vi "TCP-unpack.vi"(11 "TCP RX in":string) -> (0 "Success":bool, 1 "TCP data":string, 2 "bytecount":i32, 3 "TCP RX out (rest)":string, 5 "CountOK":bool)   [LabVIEW 2020, in "Sgraph_lib_V1.lvlib"]
uses:
  Builds/Sgraph_lib_V1.lvlib
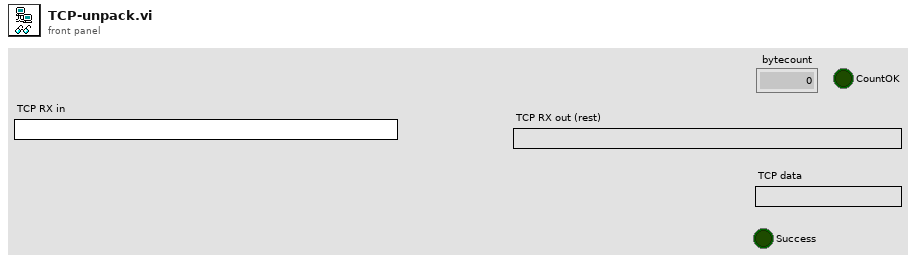
[diagram p1: front panel]
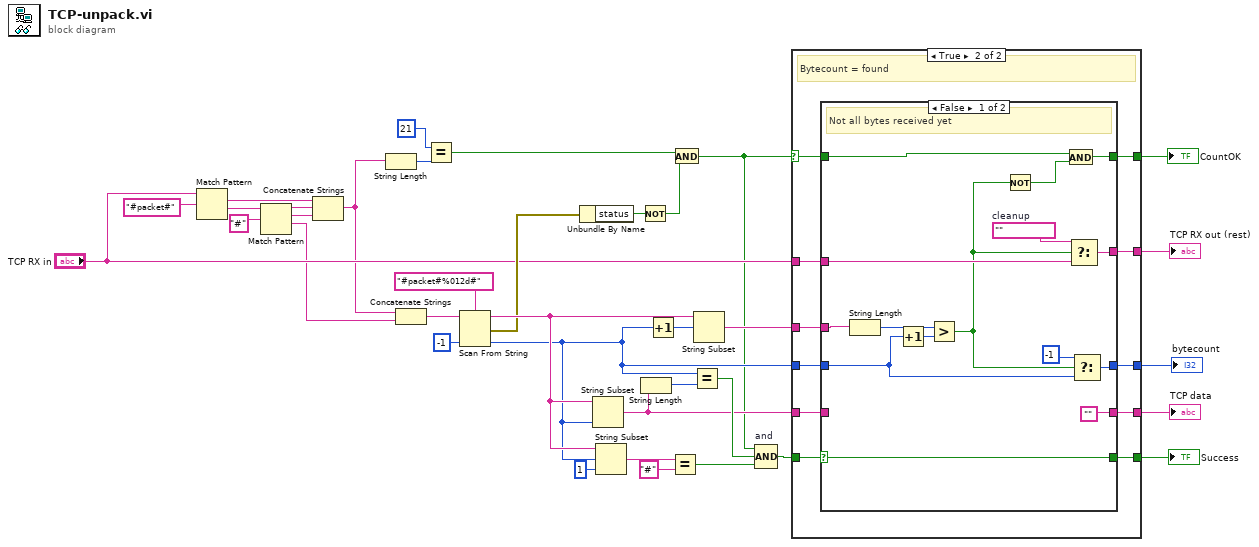
[diagram p0: block diagram]
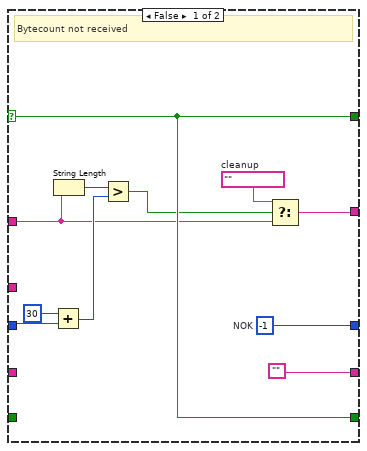
[diagram p2: hidden frame]
diagram:
  n1 = Match Pattern(string="TCP RX in", regular expression="#packet#" ("format string")) -> (match substring=w21:string, after substring=w23:string)  [unwired: 1 in, 2 out]
  n2 = Match Pattern(string=w23, regular expression="#" ("format string")) -> (before substring=w20:string, match substring=w19:string, after substring=w2:string)  [unwired: 1 in, 1 out]
  n3 = Concatenate Strings(w21, w20, w19) -> (w3:string)
  n4 = String Length(string=w3) -> (length=w18:i32)
  n5 = Concatenate Strings(w3, w2) -> (w1:string)
  n6 = Equal?(x=21, y=w18) -> (x = y?=w15:bool)
  n7 = Scan From String(format string="#packet#%012d#", input string=w1, default 1=-1 ("default value 1")) -> (remaining string=w31:string, error out=w27:errorcluster, output 1=w7:i32)  [unwired: 2 in, 1 out]
  n8 = Unbundle By Name(w27) -> ("status"=w26:bool)
  n9 = String Subset(string=w31, length (rest)=w7) -> (substring=w5:string)  [unwired: 1 in]
  n10 = String Subset(string=w31, offset (0)=w7, length (rest)=1 ("length (rest)")) -> (substring=w33:string)
  n11 = Not(x=w26) -> (.not. x?=w16:bool)
  n12 = String Length(string=w5) -> (length=w34:i32)
  n13 = Increment(x=w7) -> (x+1=w30:i32)
  n14 = Equal?(x=w33, y="#") -> (x = y?=w28:bool)
  n15 = And(x=w15, y=w16) -> (x .and. y?=w4:bool)
  n16 = Equal?(x=w7, y=w34) -> (x = y?=w29:bool)
  n17 = String Subset(string=w31, offset (0)=w30) -> (substring=w6:string)  [unwired: 1 in]
  n18 = Compound Arithmetic op=AND "and"(w4, w29, w28) -> (w8:bool)
  n19 = case shown="True" w4 {
    selector: w4 -> [w45 w49]
    tunnel: [w45 w48] -> w14
    tunnel: [w47 w52] -> w13
    tunnel: "TCP RX in" -> [w39 w56]
    tunnel: [w40 w55] -> w11
    tunnel: ["" w54] -> w10
    tunnel: [w45 w57] -> w9
    tunnel: w8 -> [_ w58]
    tunnel: w7 -> [w43 w53]
    tunnel: w6 -> [_ w51]
    tunnel: w5 -> [_ w50]
    frame False {
      w38 = ""  # cleanup
      w47 = -1  # NOK
      # "Bytecount not received"
      n20 = Add(x=30, y=w43) -> (x+y=w41:i32)
      n21 = String Length(string=w39) -> (length=w44:i32)
      n22 = Greater?(x=w44, y=w41) -> (0:w37:bool)
      n23 = Select(t=w38, s=w37, f=w39) -> (s? t:f=w40:string)
    }
    frame True {
      # "Bytecount = found"
      n24 = case shown="False" w58 {
        selector: w58 -> [w73 w78]
        tunnel: [w73 w78] -> w57
        tunnel: w56 -> [w68 _]
        tunnel: [w67 w77] -> w55
        tunnel: ["" w75] -> w54
        tunnel: w53 -> [w61 w76]
        tunnel: [w60 w76] -> w52
        tunnel: w51 -> [w71 w77]
        tunnel: w50 -> [_ w75]
        tunnel: w49 -> [w65 w74]
        tunnel: [w64 w74] -> w48
        frame False {
          w66 = ""  # cleanup
          # "Not all bytes received yet"
          n25 = String Length(string=w71) -> (length=w70:i32)
          n26 = Increment(x=w61) -> (x+1=w69:i32)
          n27 = Greater?(x=w70, y=w69) -> (0:w62:bool)
          n28 = Not(x=w62) -> (.not. x?=w63:bool)
          n29 = And(x=w65, y=w63) -> (x .and. y?=w64:bool)
          n30 = Select(t=w66, s=w62, f=w68) -> (s? t:f=w67:string)
          n31 = Select(t=-1 ("default value 1"), s=w62, f=w61) -> (s? t:f=w60:i32)
        }
        frame True {
          # "All bytes received"
        }
      }
    }
  }
  "TCP RX out (rest)" <- w11
  "TCP data" <- w10
  "Success" <- w9
  "CountOK" <- w14
  "bytecount" <- w13
